vi "Lockin.Sample.vi"(8 "error in (no error)":errorcluster, 11 "DSP in":refnum<class "DSP.lvclass">) -> (0 "error out":errorcluster, 2 "Results":T2 {"Results (Dictionary)"."value" format="%#_6p"}, 3 "DSP in":refnum<class "DSP.lvclass">)   [LabVIEW 2019, in "DSP.lvclass"]
uses:
  DSP.lvclass
  Typedefs/Results--Cluster.ctl
  Typedefs/Results Dictionary--Cluster.ctl
  DSP.lvclass/DSP.ctl
  Waveform.Attributes/Waveform.Attributes.lvlib
panel:
  out "Waveforms":T1
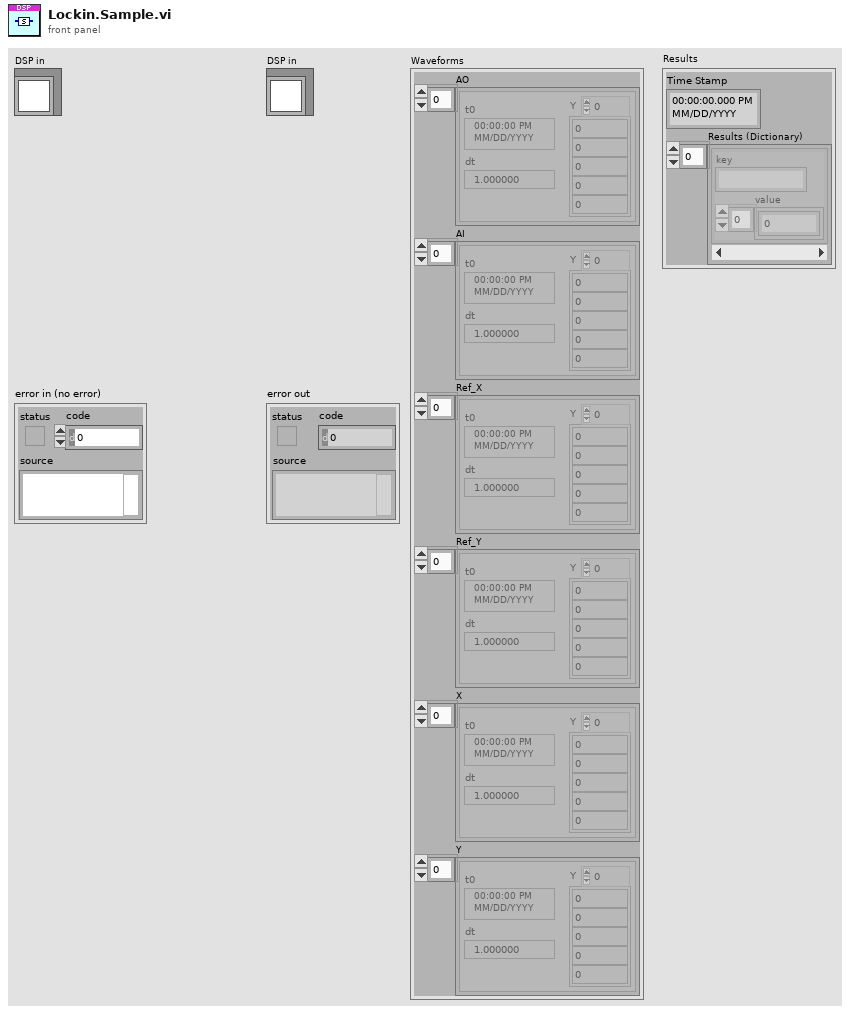
[diagram p1: front panel]
types:
  T1 = cluster{"AO":waveform(dbl)[], "AI":waveform(dbl)[], "Ref_X":waveform(dbl)[], "Ref_Y":waveform(dbl)[], "X":waveform(dbl)[], "Y":waveform(dbl)[]}
  T2 = typedef "DSP.lvclass/Results--Cluster.ctl" = cluster{"Time Stamp":timestamp, "Results (Dictionary)":T3[]}
  T3 = typedef "DSP.lvclass/Results Dictionary--Cluster.ctl" = cluster{"key":string, "value":dbl[]}
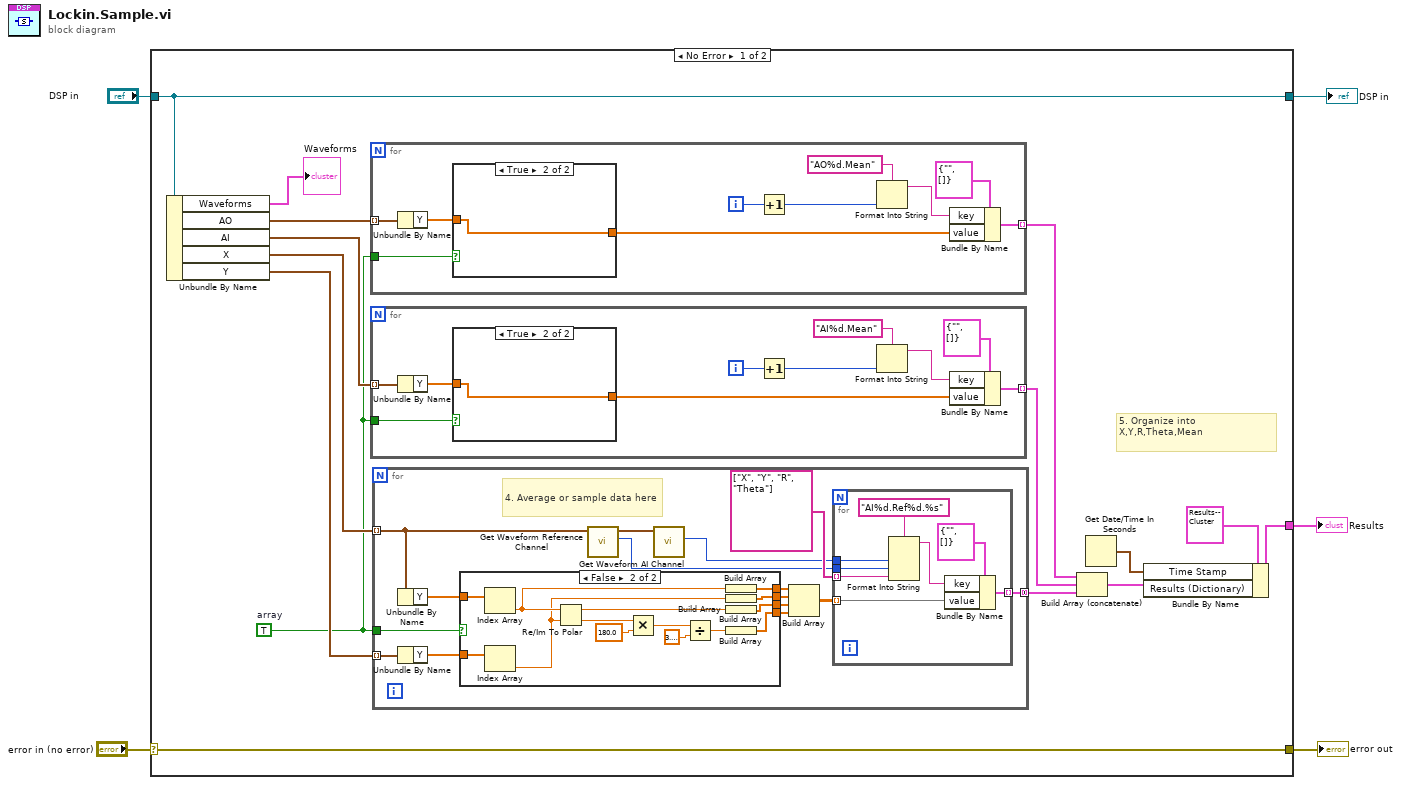
[diagram p0: block diagram]
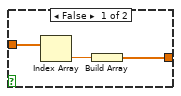
[diagram p2: hidden frame]
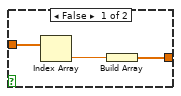
[diagram p3: hidden frame]
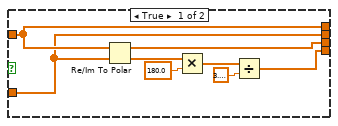
[diagram p4: hidden frame]
diagram:
  n1 = case shown="No Error" "error in (no error)" {
    selector: "error in (no error)" -> [w11 w94]
    tunnel: [w16 _] -> w5
    tunnel: [w11 w94] -> w3
    tunnel: [w10 w95] -> w2
    tunnel: "DSP in" -> [w10 w95]
    frame No Error {
      w7 = TRUE  # array
      # "5. Organize into X,Y,R,Theta,Mean"
      n2 = Unbundle By Name(w10) -> ("Waveforms"=→"Waveforms":T1, "AO"=w9:waveform(dbl)[], "AI"=w14:waveform(dbl)[], "X"=w13:waveform(dbl)[], "Y"=w12:waveform(dbl)[])
      n3 = for {
        tunnel: w9 -> [w30] mode=indexing
        tunnel: [w27] -> w15 mode=indexing
        tunnel: w7 -> [w21]
        i -> [w26]
        n4 = Unbundle By Name(w30) -> ("Y"=w22:dbl[])
        n5 = case shown="True" w21 {
          tunnel: [w31 w34] -> w24
          tunnel: w22 -> [w32 w34]
          frame False {
            n6 = Index Array(array=w32) -> (element=w33:dbl)  [unwired: 1 in]
            n7 = Build Array(w33) -> (w31:dbl[])
          }
          frame True {
          }
        }
        n8 = Increment(x=w26) -> (x+1=w25:i32)
        n9 = Format Into String(format string="AO%d.Mean", w25) -> (resulting string=w29:string)  [unwired: 2 in, 1 out]
        n10 = Bundle By Name(cluster=T3 {"key"="", "value"=[]} ("key-value"), "key"=w29, "value"=w24) -> (w27:T3)
      }
      n11 = for {
        tunnel: w14 -> [w44] mode=indexing
        tunnel: [w41] -> w18 mode=indexing
        tunnel: w7 -> [w35]
        i -> [w40]
        n12 = Unbundle By Name(w44) -> ("Y"=w37:dbl[])
        n13 = case shown="True" w35 {
          tunnel: [w45 w48] -> w36
          tunnel: w37 -> [w46 w48]
          frame False {
            n14 = Index Array(array=w46) -> (element=w47:dbl)  [unwired: 1 in]
            n15 = Build Array(w47) -> (w45:dbl[])
          }
          frame True {
          }
        }
        n16 = Increment(x=w40) -> (x+1=w39:i32)
        n17 = Format Into String(format string="AI%d.Mean", w39) -> (resulting string=w43:string)  [unwired: 2 in, 1 out]
        n18 = Bundle By Name(cluster=T3 {"key"="", "value"=[]} ("key-value"), "key"=w43, "value"=w36) -> (w41:T3)
      }
      n19 = for {
        tunnel: w13 -> [w57] mode=indexing
        tunnel: w12 -> [w60] mode=indexing
        tunnel: [w61] -> w17 mode=concatenating
        tunnel: w7 -> [w54]
        # "4. Average or sample data here"
        n20 = Unbundle By Name(w57) -> ("Y"=w63:dbl[])
        n21 = Unbundle By Name(w60) -> ("Y"=w62:dbl[])
        n22 = case shown="False" w54 {
          tunnel: w63 -> [w67 w81]
          tunnel: w62 -> [w64 w80]
          tunnel: [w67 w78] -> w53
          tunnel: [w64 w77] -> w52
          tunnel: [w66 w76] -> w51
          tunnel: [w65 w75] -> w50
          frame True {
            n23 = Re/Im To Polar(2:w64, 3:w67) -> (0:w69:dbl[], 1:w66:dbl[])
            n24 = Multiply(x=w69, y=180.0) -> (x*y=w68:dbl[])
            n25 = Divide(x=w68, y=3.141592653589793) -> (x/y=w65:dbl[])
          }
          frame False {
            n26 = Index Array(array=w81) -> (element=w79:dbl)  [unwired: 1 in]
            n27 = Index Array(array=w80) -> (element=w72:dbl)  [unwired: 1 in]
            n28 = Re/Im To Polar(2:w72, 3:w79) -> (0:w83:dbl, 1:w73:dbl)
            n29 = Multiply(x=w83, y=180.0) -> (x*y=w82:dbl)
            n30 = Divide(x=w82, y=3.141592653589793) -> (x/y=w74:dbl)
            n31 = Build Array(w79) -> (w78:dbl[])
            n32 = Build Array(w72) -> (w77:dbl[])
            n33 = Build Array(w73) -> (w76:dbl[])
            n34 = Build Array(w74) -> (w75:dbl[])
          }
        }
        n35 = call "Get Waveform Reference Channel.vi"("Reference in"=w57) -> ("Reference Channel"=w56:i32, "Reference out"=w58:waveform(dbl))  [unwired: 8 in, 1 out]
        n36 = call "Get Waveform AI Channel.vi"("Reference in"=w58) -> ("AI Channel"=w55:i32)  [unwired: 8 in, 2 out]
        n37 = Build Array(w53, w52, w51, w50) -> (w49:dbl[][])
        n38 = for {
          tunnel: w49 -> [w93] mode=indexing
          tunnel: string[] ["X", "Y", "R", "Theta"] -> [w88] mode=indexing
          tunnel: [w92] -> w61 mode=indexing
          tunnel: w56 -> [w89]
          tunnel: w55 -> [w91]
          n39 = Format Into String(format string="AI%d.Ref%d.%s", w91, w89, w88) -> (resulting string=w87:string)  [unwired: 2 in, 1 out]
          n40 = Bundle By Name(cluster=T3 {"key"="", "value"=[]} ("key-value"), "key"=w87, "value"=w93) -> (w92:T3)
        }
      }
      n41 = Build Array (concatenate)(w15, w18, w17) -> (w19:T3[])
      n42 = Get Date/Time In Seconds() -> (seconds since 1Jan1904=w20:timestamp)
      n43 = Bundle By Name(cluster=T2 {"Time Stamp"=timestamp(0 s since 1904-01-01), "Results (Dictionary)"=[]} ("Results"), "Time Stamp"=w20, "Results (Dictionary)"=w19) -> (w16:T2)
    }
    frame Error {
    }
  }
  "Results" <- w5
  "error out" <- w3
  "DSP in" <- w2
